vi "checkTimeout.vi"(8 "error in (no error)":errorcluster, 10 "executionTime":u32, 11 "TCPClient in":refnum<class "TCPClient.lvclass">) -> (0 "error out":errorcluster, 3 "TCPClient out":refnum<class "TCPClient.lvclass">)   [LabVIEW 2016, in "tcp.lvlib" / "TCPClient.lvclass"]
uses:
  TCPClient.lvclass
  TCPClient.lvclass/TCPClient.ctl
panel:
  out "timeout":bool
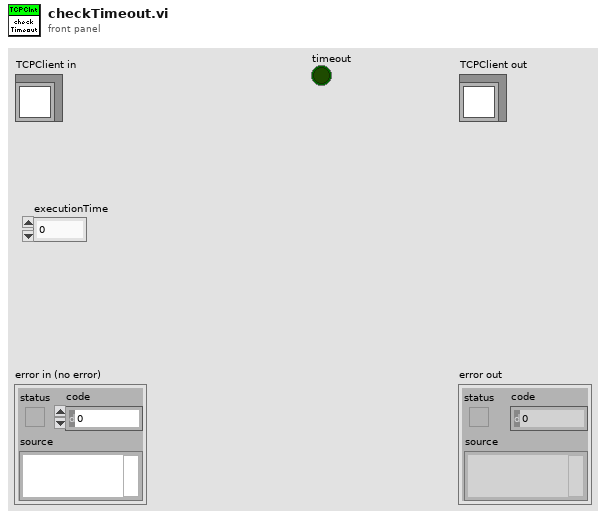
[diagram p1: front panel]
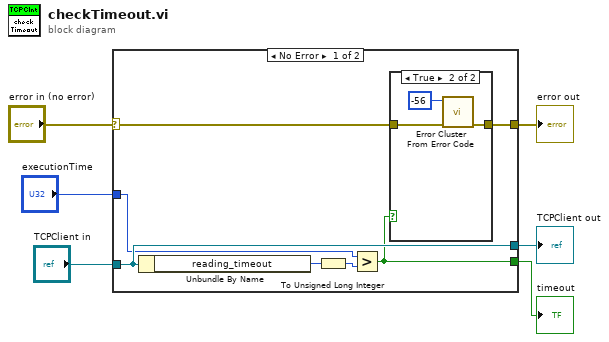
[diagram p0: block diagram]
diagram:
  n1 = case shown="No Error" "error in (no error)" {
    selector: "error in (no error)" -> [w9 w19]
    tunnel: [w7 w19] -> w5
    tunnel: [w12 w18] -> w3
    tunnel: "TCPClient in" -> [w12 w18]
    tunnel: "executionTime" -> [w10 _]
    tunnel: [w8 _] -> w1
    frame No Error {
      n2 = Unbundle By Name(w12) -> ("reading_timeout"=w13:i32)
      n3 = To Unsigned Long Integer(number=w13) -> (unsigned 32bit integer=w11:u32)
      n4 = Greater?(x=w10, y=w11) -> (0:w8:bool)
      n5 = case shown="True" w8 {
        tunnel: w9 -> [w14 w17]
        tunnel: [w14 w16] -> w7
        frame False {
        }
        frame True {
          n6 = call <vilib>:"Error Cluster From Error Code.vi"("error in (no error)"=w17, "error code (0)"=-56) -> ("error out"=w16:errorcluster)  [unwired: 7 in]
        }
      }
    }
    frame Error {
    }
  }
  "error out" <- w5
  "TCPClient out" <- w3
  "timeout" <- w1
